vi "VAT_valve_get_unit.vi"(0 "VAT Valve COM port":refnum<visa-resource-name>, 11 "error in (no error)":errorcluster) -> (4 "VAT Valve COM port out":refnum<visa-resource-name>, 13 "Unit":string, 15 "error out":errorcluster)   [LabVIEW 2019]
uses:
  <vilib>/regexp/Match Regular Expression.xnode
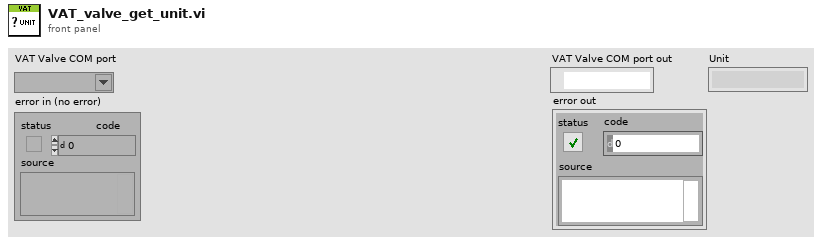
[diagram p1: front panel]
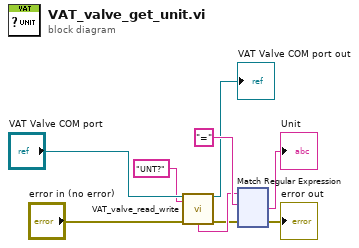
[diagram p0: block diagram]
diagram:
  n1 = call "VAT_valve_read_write.vi"("VAT Valve COM port"="VAT Valve COM port", "Write String"="UNT?", "error in (no error)"="error in (no error)") -> ("VAT Valve COM port out"=→"VAT Valve COM port out":refnum<visa-resource-name>, "Read String"=w3:string, "error out"=w1:errorcluster)  [unwired: 10 in]
  n2 = xnode "Match Regular Expression"("input string"=w3, "regular expression"="=" ("search string/char (-)"), "error in"=w1) -> ("after match"=→"Unit":string, "error out"=→"error out":errorcluster)  [unwired: 3 in, 3 out]
